vi "cp.vi"(0 "IP adress":string="192.109.209.229", 1 "stop":bool, 2 "Channel":u8(ring) items=["1", "2", "3", "4", "5", "6", "7", "8", "9", "10", "11", "12", "13", "14", "15", "16"], 3 "CP Parameters":T1={"Steps"=[{"vs_initial"=FALSE, "Current_step"=0.0, "Duration_step"=1.0}, {"vs_initial"=FALSE, "Current_step"=0.001, "Duration_step"=1.0}, {"vs_initial"=FALSE, "Current_step"=0.005, "Duration_step"=1.0}], "Step_number"=2, "N_Cycles"=0, "Record_every_dE"=0.005, "Record_every_dT"=0.05, "I_Range"=8, "E_Range"=3, "Bandwidth"=5, "em"=1, "ce"=0, "tb"=2.5e-05} {"tb" min=2.5e-05 max=1 format="%^_3e"; "ce" items=["Standard", "CE to ground"]; "N_Cycles" min=0 max=1000000; "Step_number" min=0 max=99; "E_Range" items=["±2.5V", "±5V", "±10V", "Auto"]; "Bandwidth" items=["1"=1, "2"=2, "3"=3, "4"=4, "5"=5, "6"=6, "7"=7, "8"=8, "9"=9]; "Record_every_dT" min=0.0001 max=1000 format="%^_3e"; "Record_every_dE" format="%^_3e"; "I_Range" items=["1pA", "1nA", "10nA", "100nA", "1µA", "10µA", "100µA", "1mA", "10mA", "100mA", "1A", "Booster"]; "Steps"."Duration_step" min=0.001 max=80000 format="%^_3e"; "Steps"."Current_step" min=-150 max=150 format="%^_3e"}, 4 "Exit":bool, 5 "Start":bool, 6 "Draw":enum16{"Ewe(t)", "I(t)"}(ring)) -> (7 "XY Graph":cluster{"Data 101":sgl[], "Data 101":sgl[]}(graph), 8 "Number of points":i32=5992)   [LabVIEW 2016]
doc: "The Chrono-Potentiometry (CP) is a controlled current technique. The current is controlled and the potential is the variable determined as a function of time.\nIn general, in this VI, the first thing to do is to start by establishing the connection with the instrument defined by its IP adress, then load the firmware in the channel selected, get the information on the plugged channels, load protocol on a channel, start/stop the protocol, retreive data and draw the graph."
uses:
  LLB/dll_Functions.llb/CPParameters.ctl
panel:
  in  "Display Parameters?":bool caption="Display Parameters"
  out "DllPath":path caption="DLL Path"
  out "LibVersion":string caption="DLL Version"
  out "Exit 2":bool=TRUE
  out "Data 102":sgl[][](array[numeric]) format="%.2f"
  # "Instructions:\nBefore running the VI you must type a valid IP adress that corresponds to the instrument.Then press the Run button to execute this VI.\nWhile this VI is running, choose the available channel, enter the CP parameters or keep the default values, then press the start button to begin the experience.\nChoose the waveform to draw (Ewe(t) or I(t)). You can stop the measure if you press the stop button and exit the execution if you press the exit button."
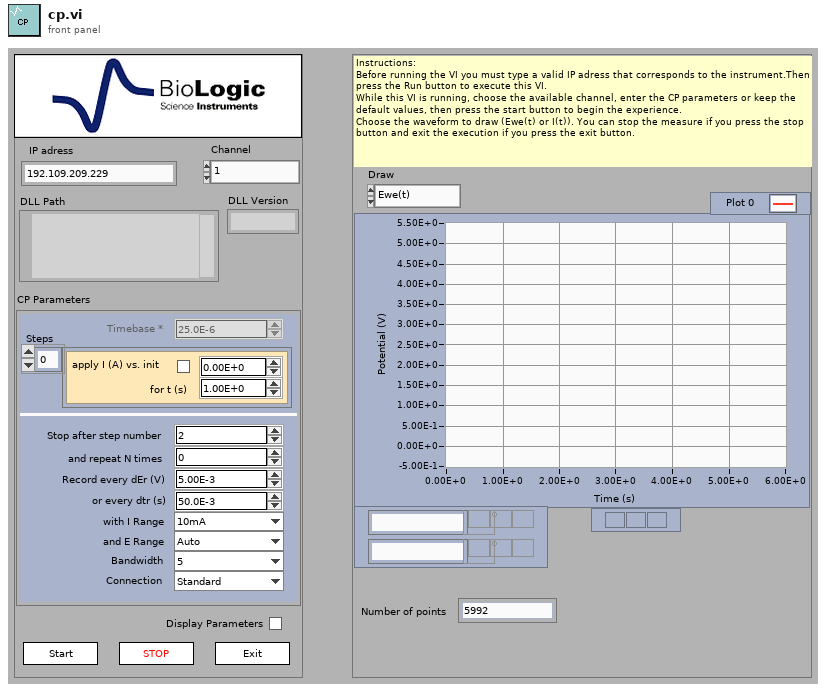
[diagram p1: front panel]
types:
  T1 = typedef "CPParameters.ctl" = cluster{"Steps":cluster{"vs_initial":bool, "Current_step":sgl, "Duration_step":sgl}[], "Step_number":i32, "N_Cycles":i32, "Record_every_dE":sgl, "Record_every_dT":sgl, "I_Range":u16, "E_Range":u16, "Bandwidth":u16, "em":u16, "ce":u16, "tb":sgl}
  T2 = cluster{"LibVersion":string, "StringLength":u32, "DllPath":path}
  T3 = cluster{"Channel":i32, "BoardVersion":i32, "BoardSerialCode":i32, "FirmwareCode":i32, "FirmwareVersion":i32, "XilinxVersion":i32, "AmpCode":i32, "NbAmp":i32, "LcBoard":i32, "Zboard":i32, "MuxBoard":i32, "GPRAboard":i32, "MemSize":i32, "MemFilled":i32, "state":i32, "MaxIRange":i32, "MinIRange":i32, "MaxBandwidth":i32, "NbOfTechniques":i32}
  T4 = typedef "TechniqueParameters.ctl" = cluster{"String Label":string, "Type":i32, "Valeur":i32, "Index":i32}
  T5 = cluster{"string before end tag":string, i32, i32, i32}[]
  T6 = cluster{"IRQskipped":i32, "NbRaws":i32, "NbCols":i32, "Technique Index":i32, "TechniqueID":i32, "PrcessIndex":i32, "loop":i32, "StartTime":dbl, "MuxPad":i32}
  T7 = cluster{"State":i32, "MemFilled":i32, "TimeBase":sgl, " Ewe":sgl, " EweRangeMin":sgl, " EweRangeMax":sgl, "Ece":sgl, "EceRangeMin":sgl, "EceRangeMax":sgl, "Eoverflow":i32, "I":sgl, "IRange":i32, "Ioverflow":i32, "ElapsedTime":sgl, "Freq":sgl, "Rcomp":sgl, "Saturation":sgl, "OptErr":i32, "OptPos":i32}
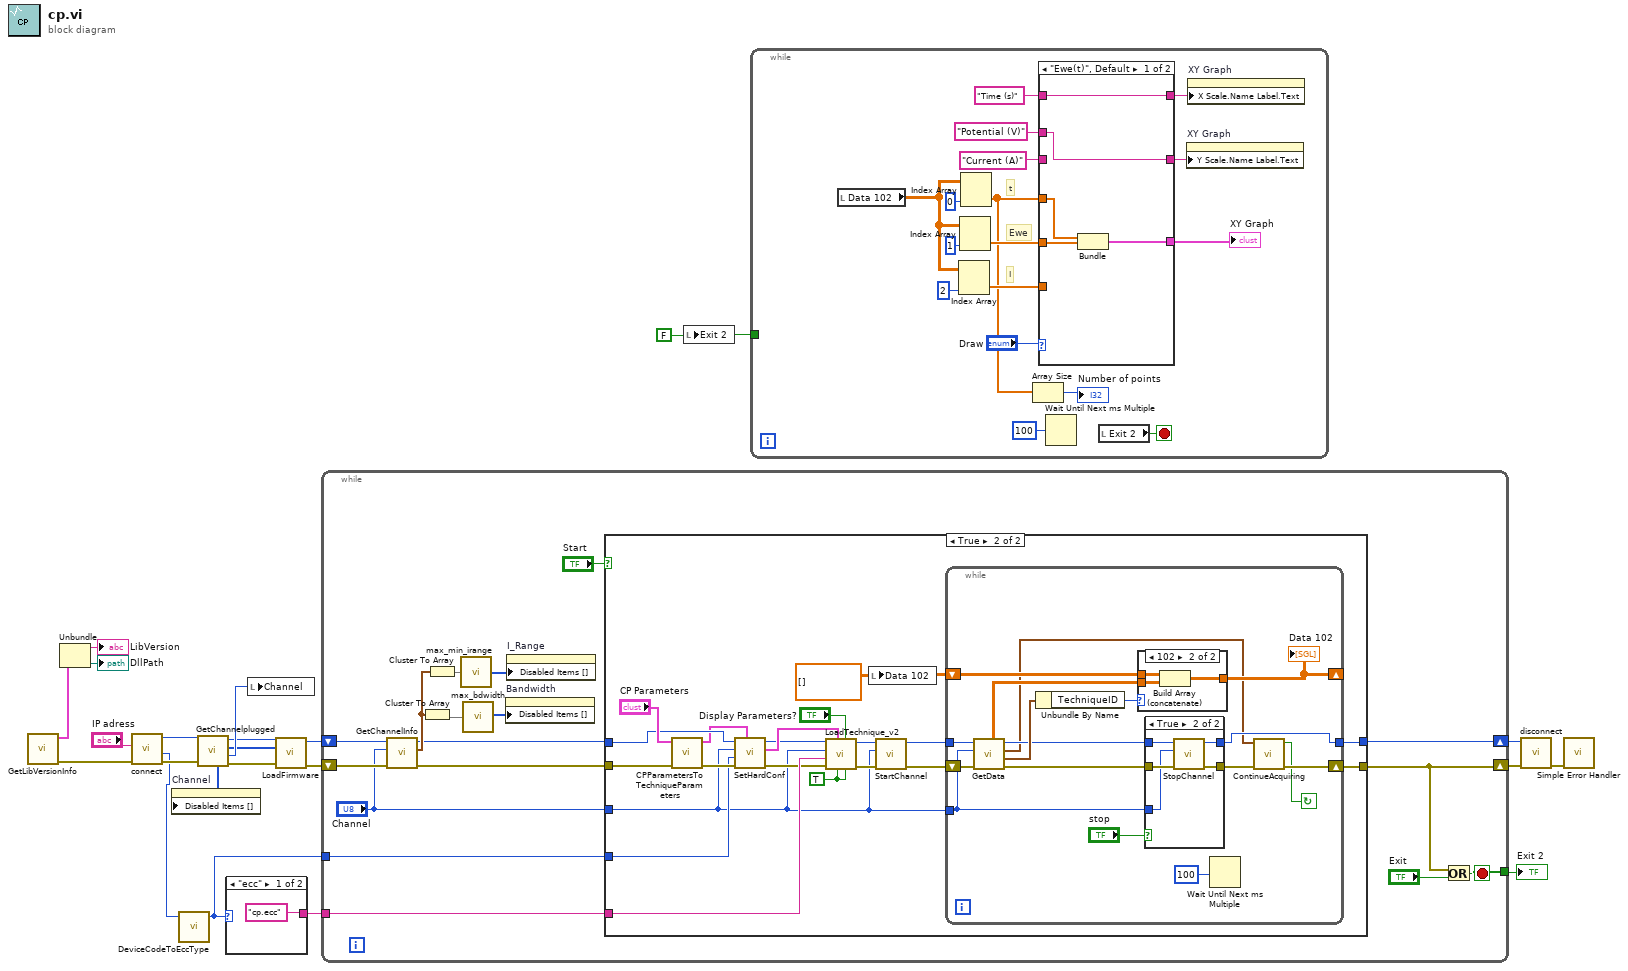
[diagram p0: block diagram]
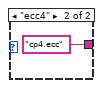
[diagram p2: hidden frame]
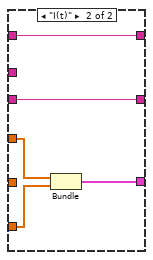
[diagram p3: hidden frame]
diagram:
  w21 = FALSE ("Exit 2")
  n1 = call "GetLibVersionInfo.vi"() -> ("error out"=w1:errorcluster, "LibInfo"=w4:T2)  [unwired: 10 in]
  n2 = Unbundle(w4) -> ("LibVersion"=→"LibVersion":string, "DllPath"=→"DllPath":path)  [unwired: 1 out]
  n3 = call "connect.vi"("error in (no error)"=w1, "IP"="IP adress") -> ("error out"=w17:errorcluster, "Device Code"=w8:i32, "ID Out"=w13:i32)  [unwired: 6 in, 1 out]
  n4 = call "DeviceCodeToEccType.vi"("Device Code"=w8) -> ("EccType"=w5:enum16{"ecc", "ecc4"})  [unwired: 4 in]
  n5 = call "GetChannelplugged.vi"("error in (no error)"=w17, "ID In"=w13) -> ("error out"=w16:errorcluster, "FirstPluggedChannel"=w19:u8, "PluggedChannels"=w10:u8[], "ID Out"=w14:i32, "DisabledChannels"=w11:i32[])  [unwired: 5 in]
  n6 = property on="Channel" class="Ring (strict)"("Disabled Items []"=w11) -> ()  [unwired: 2 in, 2 out]
  n7 = case shown="\"ecc\"" w5 {
    tunnel: ["cp.ecc" ("FName") "cp4.ecc" ("FName4")] -> w7
    frame "ecc" {
    }
    frame "ecc4" {
    }
  }
  n8 = local write "Channel"(w19) -> ()
  n9 = call "LoadFirmware.vi"("error in (no error)"=w16, "Channels"=w10, "ID In"=w14) -> ("error out"=w15:errorcluster, "ID Out"=w12:i32)  [unwired: 6 in, 1 out]
  n10 = while {
    shift-right: [w28] -> w9
    shift-left: w15 -> [w35]
    tunnel: [w26] -> w22
    shift-right: [w38] -> w18
    shift-left: w12 -> [w31]
    tunnel: w7 -> [w29]
    tunnel: w5 -> [w25]
    stop <- w26 stop-if-true
    n11 = call "GetChannelInfo.vi"("error in (no error)"=w35, "Channel"="Channel", "ID"=w31) -> ("error out"=w33:errorcluster, "Channel information"=w32:T3, "ID Out"=w30:i32)  [unwired: 6 in]
    n12 = Cluster To Array(cluster=w32) -> (array=w39:i32[])
    n13 = Cluster To Array(cluster=w32) -> (array=w40:i32[])
    n14 = call "max_min_irange.vi"("resources"=w40) -> ("disabled ranges"=w37:i32[])
    n15 = call "max_bdwidth.vi"("resources"=w39) -> ("disabled ranges"=w36:i32[])
    n16 = property on="Bandwidth" class="Ring (strict)"("Disabled Items []"=w36) -> ()  [unwired: 2 in, 2 out]
    n17 = property on="I_Range" class="Ring (strict)"("Disabled Items []"=w37) -> ()  [unwired: 2 in, 2 out]
    n18 = case shown="True" "Start" {
      tunnel: "Channel" -> [_ w45]
      tunnel: [w43 w63] -> w28
      tunnel: w33 -> [w43 w53]
      tunnel: w30 -> [w42 w51]
      tunnel: [w42 w54] -> w38
      tunnel: w29 -> [_ w56]
      tunnel: w25 -> [_ w46]
      frame False {
      }
      frame True {
        w55 = TRUE ("First Protocol")
        w62 = sgl[][] []
        n19 = call "CPParametersToTechniqueParameters.vi"("error in (no error)"=w53, "CP Parameters"="CP Parameters") -> ("error out"=w52:errorcluster, "TechniqueParameters"=w50:T4[])  [unwired: 8 in]
        n20 = call "SetHardConf.vi"("Params Values"=w50, "error in (no error)"=w52, "EccType"=w46, "Channel"=w45, "ID In"=w51) -> ("error out"=w47:errorcluster, "Params Values Trimed"=w49:T5, "ID Out"=w48:i32)  [unwired: 4 in]
        n21 = call "LoadTechnique_v2.vi"("Last Protocol"=w55, "Display Parameters?"="Display Parameters?", "First Protocol"=w55, "TechniqueParameters"=w49, "error in (no error)"=w47, "FName"=w56, "Selected Channel"=w45, "ID In"=w48) -> ("error out"=w59:errorcluster, "ID  Out"=w58:i32)  [unwired: 2 in]
        n22 = local write "Data 102"(w62) -> ()
        n23 = call "StartChannel.vi"("error in (no error)"=w59, "Channel"=w45, "ID In"=w58) -> ("error out"=w60:errorcluster, "ID Out"=w57:i32)  [unwired: 7 in]
        n24 = while {
          shift-right: [w67] -> w63
          shift-left: w60 -> [w80]
          shift-right: [w77] -> _
          shift-left: w62 -> [w78]
          tunnel: w45 -> [w69]
          tunnel: w57 -> [w75]
          tunnel: [w70] -> w54
          stop <- w65 continue-if-true
          n25 = call "GetData.vi"("error in (no error)"=w80, "Channel"=w69, "ID In"=w75) -> ("error out"=w68:errorcluster, "Data information"=w74:T6, "Current values"=w64:T7, "ID Out"=w71:i32, "Data"=w72:dbl[][])  [unwired: 4 in]
          n26 = Unbundle By Name(w74) -> ("TechniqueID"=w73:i32)
          n27 = case shown="102" w73 {
            tunnel: w72 -> [_ w91]
            tunnel: w78 -> [w88 w90]
            tunnel: [w88 w89] -> w77
            frame 0, Default {
            }
            frame 102 {
              n28 = Build Array (concatenate)(w90, w91) -> (w89:dbl[][])
            }
          }
          "Data 102" <- w77
          n29 = case shown="True" "stop" {
            tunnel: [w82 w87] -> w66
            tunnel: w68 -> [w82 w86]
            tunnel: w71 -> [w81 w85]
            tunnel: [w81 w84] -> w70
            tunnel: w69 -> [_ w83]
            frame False {
            }
            frame True {
              n30 = call "StopChannel.vi"("error in (no error)"=w86, "Channel"=w83, "ID In"=w85) -> ("error out"=w87:errorcluster, "ID Out"=w84:i32)  [unwired: 7 in]
            }
          }
          n31 = Wait Until Next ms Multiple(millisecond multiple=u32 100) -> ()  [unwired: 1 out]
          n32 = call "ContinueAcquiring.vi"("error in"=w66, "Current values"=w64) -> ("error out"=w67:errorcluster, "ContinueAcquiring?"=w65:bool)  [unwired: 8 in]
        }
      }
    }
    n33 = Or(x=w28, y="Exit") -> (x .or. y?=w26:bool)
  }
  "Exit 2" <- w22
  n34 = local write "Exit 2"(w21) -> ()
  n35 = while {
    tunnel: w21 -> [_]
    stop <- w107 stop-if-true
    # "I"
    # "Ewe"
    # "t"
    n36 = local read "Data 102"() -> (w96:sgl[][])
    n37 = Index Array(array=w96, index (col)=2 ("indice désactivé (col)")) -> (element=w93:sgl[])  [unwired: 1 in]
    n38 = Index Array(array=w96, index (col)=1 ("Index")) -> (element=w95:sgl[])  [unwired: 1 in]
    n39 = Index Array(array=w96, index (col)=0 ("Index")) -> (element=w92:sgl[])  [unwired: 1 in]
    n40 = Array Size(array=w92) -> (size(s)=→"Number of points":i32)
    n41 = case shown="\"Ewe(t)\", Default" "Draw" {
      tunnel: w92 -> [w113 w118]
      tunnel: [w110 w114] -> w94
      tunnel: "Potential (V)" ("Y Scale.Name Label.Text") -> [w112 _]
      tunnel: "Current (A)" ("Y Scale.Name Label.Text") -> [_ w117]
      tunnel: [w112 w117] -> w101
      tunnel: [w111 w116] -> w100
      tunnel: "Time (s)" ("Y Scale.Name Label.Text") -> [w111 w116]
      tunnel: w95 -> [w109 _]
      tunnel: w93 -> [_ w115]
      frame "Ewe(t)", Default {
        n42 = Bundle("Data 102"=w113, "Data 102"=w109) -> (w110:cluster{"Data 102":sgl[], "Data 102":sgl[]})  [unwired: 1 in]
      }
      frame "I(t)" {
        n43 = Bundle("Data 102"=w118, "Data 102"=w115) -> (w114:cluster{"Data 102":sgl[], "Data 102":sgl[]})  [unwired: 1 in]
      }
    }
    "XY Graph" <- w94
    n44 = Wait Until Next ms Multiple(millisecond multiple=u32 100) -> ()  [unwired: 1 out]
    n45 = local read "Exit 2"() -> (w107:bool)
    n46 = property on="XY Graph" class="XYGraph (strict)"("Y Scale.Name Label.Text"=w101) -> ()  [unwired: 2 in, 2 out]
    n47 = property on="XY Graph" class="XYGraph (strict)"("X Scale.Name Label.Text"=w100) -> ()  [unwired: 2 in, 2 out]
  }
  n48 = call "disconnect.vi"("error in (no error)"=w9, "ID In"=w18) -> ("error out"=w6:errorcluster)  [unwired: 9 in]
  n49 = call <vilib>:"Simple Error Handler.vi"("error in (no error)"=w6) -> ()  [unwired: 4 in, 5 out]
